vi "Test Xiaolei Hu.vi"() -> ()   [LabVIEW 2017]
doc: "Created IvanLis by LabVIEW Portal\nProfile: http://labviewportal.org/memberlist.php?mode=viewprofile&u=987\neMail: IvanLisanov@gMail.com\nTelegram: https://t.me/IvanLis"
uses:
  libonnx_wrapper/libonnx_wrapper.lvlib
  libonnx_wrapper/TypeDef/IO.ctl
  libonnx_wrapper/TypeDef/Introspection.ctl
panel:
  in  "threshold":sgl=0.3 format="%#.6g"
  in  "max Object's":i64=9
  in  "Tab Control":enum32{"Result", "Introspection"}(tab)
  out "detected_boxes":sgl[][](array[numeric])
  out "detected_classes":sgl[](array[numeric])
  out "score":sgl[](array[numeric])
  out "Introspection Input":T1
  out "Introspection Output":T1
  out "2D Picture":picture
  out "PNG file path":path=path "/home/ivan/LabVIEWData/ONNX/LabVIEW-ONNX_Runtime/image_for_test/1_1_2r_1_1_var10.jpg"
  out "ONNX model path":path=path "/home/ivan/LabVIEWData/ONNX/LabVIEW-ONNX_Runtime/data/coins_detection.onnx"
  out "error out":errorcluster
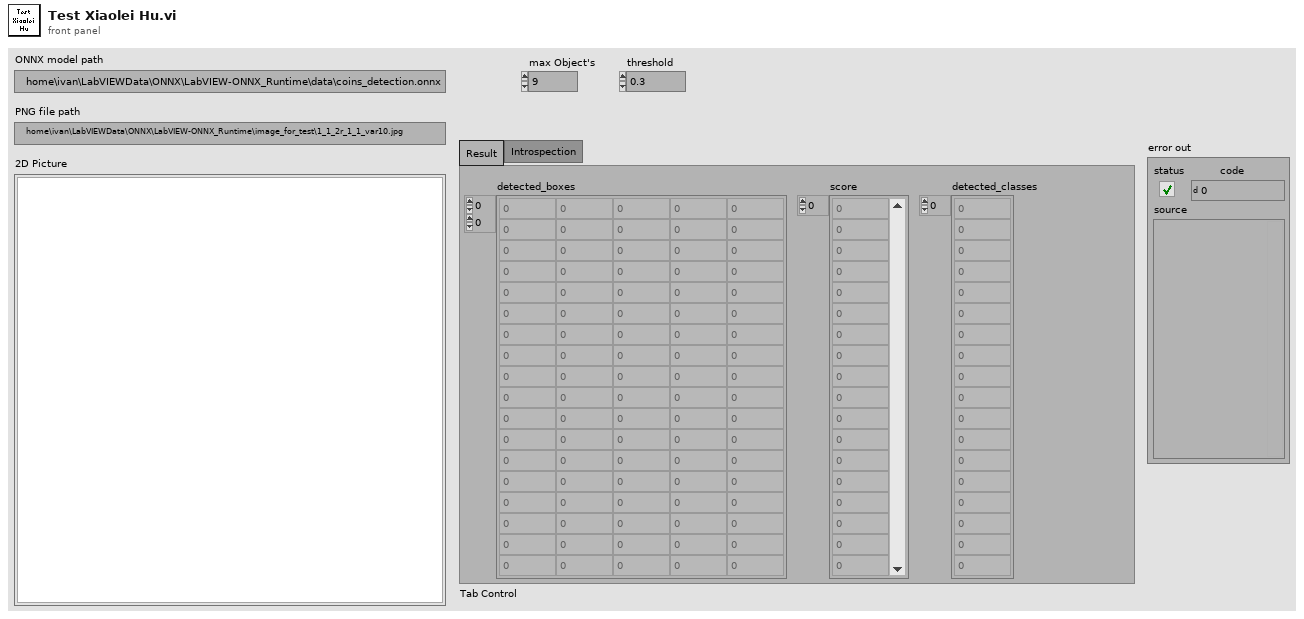
[diagram p1: front panel]
types:
  T1 = typedef "libonnx_wrapper.lvlib/Introspection.ctl" = cluster{"Count":i32, "Shapes":T2[]}
  T2 = typedef "libonnx_wrapper.lvlib/IO.ctl" = cluster{"Name":string, "DimCount":i32, "Type Index":i32, "Type Name":string, "Dims":i64[]}
  T3 = typedef "imagedata.ctl" = cluster{"image type":i32, "image depth":i32, "image":u8[], "mask":u8[], "colors":u32[], "Rectangle":cluster{"left":i16, "top":i16, "right":i16, "bottom":i16}}
  T4 = cluster{"left":i16, "top":i16, "right":i16, "bottom":i16}
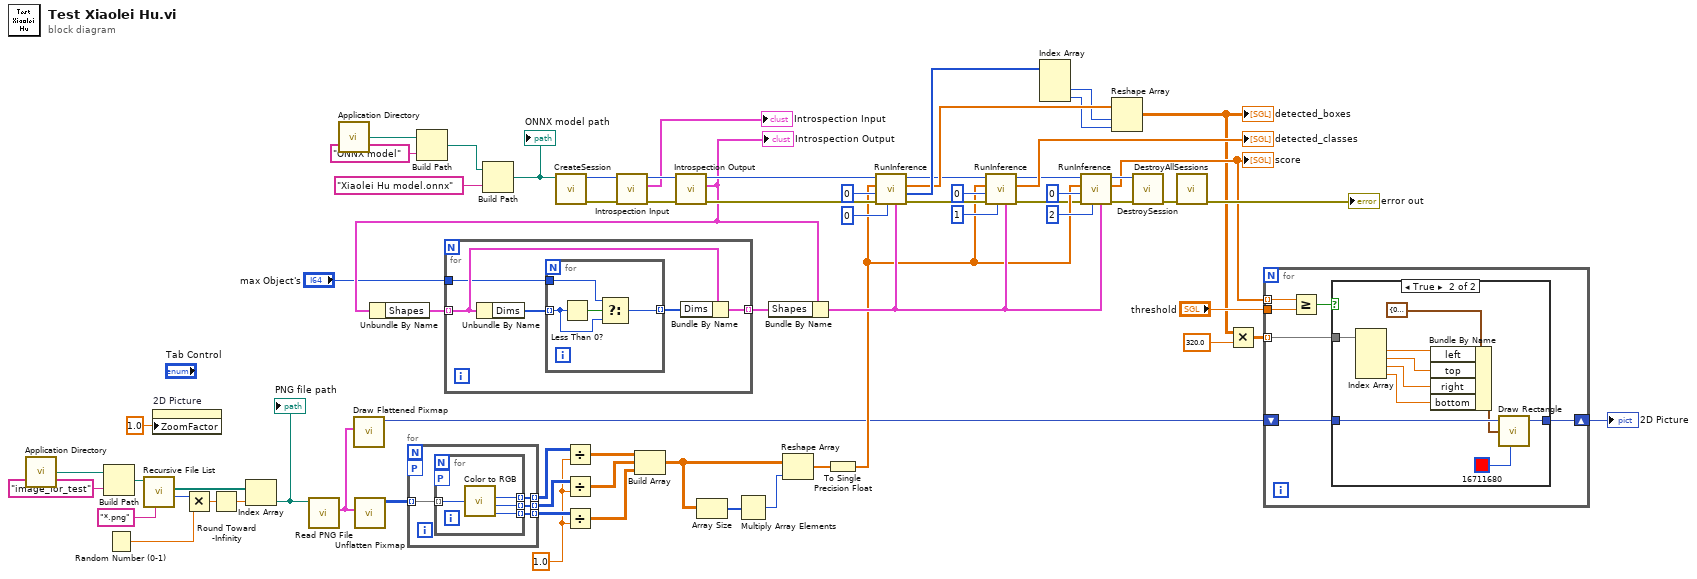
[diagram p0: block diagram]
diagram:
  w51 = 1.0 ("y")
  n1 = call <vilib>:"Application Directory.vi"() -> ("Application Directory"=w17:path)
  n2 = Build Path(base path=w17, name or relative path="image_for_test") -> (appended path=w16:path)
  n3 = Random Number (0-1)() -> (number: 0 to 1=w14:dbl)
  n4 = call <vilib>:"Recursive File List.vi"("pattern"="*.png", "Folder Path"=w16) -> ("Number of Files"=w13:i32, "All Files in Dir"=w11:path[])  [unwired: 5 in, 3 out]
  n5 = property on="2D Picture" class="Pict"("ZoomFactor"=sgl 1.0 ("Zoom Factor")) -> ()  [unwired: 2 in, 2 out]
  n6 = Multiply(x=w13, y=w14) -> (x*y=w12:dbl)
  n7 = Round Toward -Infinity(1:w12) -> (0:w10:dbl)
  n8 = Index Array(array=w11, index=w10) -> (element=w9:path)
  "PNG file path" <- w9
  n9 = call <vilib>:"Read PNG File.vi"("path to PNG file"=w9) -> ("image data"=w50:T3)  [unwired: 8 in, 2 out]
  n10 = call <vilib>:"Application Directory.vi"() -> ("Application Directory"=w65:path)
  n11 = call <vilib>:"Draw Flattened Pixmap.vi"("image data"=w50) -> ("new picture"=w7:picture)  [unwired: 8 in]
  n12 = call <vilib>:"Unflatten Pixmap.vi"("image data"=w50) -> ("24-bit pixmap"=w62:u32[][])  [unwired: 10 out]
  n13 = for {
    tunnel: w62 -> [w72] mode=indexing
    tunnel: [w71] -> w52 mode=indexing
    tunnel: [w70] -> w53 mode=indexing
    tunnel: [w69] -> w54 mode=indexing
    workers-P: _ -> [_]
    n14 = for {
      tunnel: w72 -> [w73] mode=indexing
      tunnel: [w76] -> w71 mode=indexing
      tunnel: [w75] -> w70 mode=indexing
      tunnel: [w74] -> w69 mode=indexing
      workers-P: _ -> [_]
      n15 = call <vilib>:"Color to RGB.vi"("Color"=w73) -> ("R"=w76:u8, "G"=w75:u8, "B"=w74:u8)  [unwired: 1 out]
    }
  }
  n16 = Build Path(base path=w65, name or relative path="ONNX model") -> (appended path=w63:path)
  n17 = Build Path(base path=w63, name or relative path="Xiaolei Hu model.onnx") -> (appended path=w66:path)
  "ONNX model path" <- w66
  n18 = call "CreateSession.vi"("ONNX model path"=w66) -> ("error out"=w44:errorcluster, "session id out"=w45:i32)  [unwired: 9 in]
  n19 = Divide(x=w52, y=w51) -> (x/y=w55:dbl[][])
  n20 = Divide(x=w53, y=w51) -> (x/y=w56:dbl[][])
  n21 = Divide(x=w54, y=w51) -> (x/y=w57:dbl[][])
  n22 = call "Introspection Input.vi"("error in (no error)"=w44, "session id in"=w45) -> ("error out"=w47:errorcluster, "Introspection Input"=→"Introspection Input":T1, "session id out"=w48:i32)  [unwired: 7 in]
  n23 = Build Array(w55, w56, w57) -> (w59:dbl[][][])
  n24 = call "Introspection Output.vi"("error in (no error)"=w47, "session id in"=w48) -> ("error out"=w39:errorcluster, "Introspection Output"=w37:T1, "session id out"=w40:i32)  [unwired: 7 in]
  "Introspection Output" <- w37
  n25 = Unbundle By Name(w37) -> ("Shapes"=w41:T2[])
  n26 = for {
    tunnel: w41 -> [w80] mode=indexing
    tunnel: [w78] -> w38 mode=indexing
    tunnel: "max Object's" -> [w77]
    n27 = Unbundle By Name(w80) -> ("Dims"=w81:i64[])
    n28 = for {
      tunnel: w81 -> [w84] mode=indexing
      tunnel: [w83] -> w79 mode=indexing
      tunnel: w77 -> [w82]
      n29 = Less Than 0?(x=w84) -> (x < 0?=w85:bool)
      n30 = Select(t=w82, s=w85, f=w84) -> (s? t:f=w83:i64)
    }
    n31 = Bundle By Name(cluster=w80, "Dims"=w79) -> (w78:T2)
  }
  n32 = Array Size(array=w59) -> (size(s)=w58:i32[])
  n33 = Multiply Array Elements(1:w58) -> (0:w60:i32)
  n34 = Bundle By Name(cluster=w37, "Shapes"=w38) -> (w21:T1)
  n35 = Reshape Array(w59, w60) -> (w61:dbl[])
  n36 = To Single Precision Float(number=w61) -> (single precision float=w20:sgl[])
  n37 = call "RunInference.vi"("Introspection Output"=w21, "outputIndex"=0, "error in (no error)"=w39, "inputIndex"=0, "inputBuffer"=w20, "session id in"=w40) -> ("error out"=w28:errorcluster, "Dims"=w35:i64[], "outputBuffer"=w34:sgl[], "session id out"=w30:i32)  [unwired: 2 in]
  n38 = call "RunInference.vi"("Introspection Output"=w21, "outputIndex"=1, "error in (no error)"=w28, "inputIndex"=0, "inputBuffer"=w20, "session id in"=w30) -> ("error out"=w19:errorcluster, "outputBuffer"=→"detected_classes":sgl[], "session id out"=w22:i32)  [unwired: 2 in, 1 out]
  n39 = Index Array(array=w35) -> (element #2=w33:i64, element #3=w32:i64)  [unwired: 3 in, 1 out]
  n40 = call "RunInference.vi"("Introspection Output"=w21, "outputIndex"=2, "error in (no error)"=w19, "inputIndex"=0, "inputBuffer"=w20, "session id in"=w22) -> ("error out"=w24:errorcluster, "outputBuffer"=w8:sgl[], "session id out"=w23:i32)  [unwired: 2 in, 1 out]
  "score" <- w8
  n41 = Reshape Array(w34, w33, w32) -> (w4:sgl[][])
  "detected_boxes" <- w4
  n42 = call "DestroySession.vi"("error in (no error)"=w24, "session id in"=w23) -> ("error out"=w49:errorcluster)  [unwired: 8 in, 1 out]
  n43 = call "DestroyAllSessions.vi"("error in (no error)"=w49) -> ("error out"=→"error out":errorcluster)  [unwired: 10 in]
  n44 = Multiply(x=w4, y=sgl 320.0) -> (x*y=w3:sgl[][])
  n45 = for {
    tunnel: w8 -> [w91] mode=indexing
    shift-right: [w86] -> w2
    shift-left: w7 -> [w88]
    tunnel: "threshold" -> [w90]
    tunnel: w3 -> [w87] mode=indexing
    n46 = Greater Or Equal?(x=w91, y=w90) -> (x >= y?=w89:bool)
    n47 = case shown="True" w89 {
      tunnel: w88 -> [w92 w102]
      tunnel: w87 -> [_ w101]
      tunnel: [w92 w100] -> w86
      frame False {
      }
      frame True {
        n48 = Index Array(array=w101) -> (element #1=w96:sgl, element #2=w95:sgl, element #3=w94:sgl, element #4=w93:sgl)  [unwired: 4 in]
        n49 = Bundle By Name(cluster=T4 {"left"=0, "top"=0, "right"=0, "bottom"=0} ("rect"), "left"=w96, "top"=w95, "right"=w94, "bottom"=w93) -> (w97:T4)
        n50 = call <vilib>:"Draw Rectangle.vi"("picture"=w102, "rect"=w97, "color(black)"=u32 16711680) -> ("new picture"=w100:picture)  [unwired: 6 in]
      }
    }
  }
  "2D Picture" <- w2
